vi "CS-4 Get Rates.vi"(6 "error in (no error)":errorcluster, 9 "VISA session":refnum<visa-resource-name>) -> (0 "error out":errorcluster, 2 "sweep rates":T1={"rate 0"=0.5, "rate 1"=0.25, "rate 2"=0.1, "rate 3"=10.0} {"rate 3" min=0.0 max=100.0 step=1.0 format="%.4f"; "rate 2" min=0.0 max=100.0 step=0.05 format="%.4f"; "rate 1" min=0.0 max=100.0 step=0.05 format="%.4f"; "rate 0" min=0.0 max=100.0 step=0.05 format="%.4f"}, 3 "dup VISA session":refnum<visa-resource-name>)   [LabVIEW 2016]
doc: "CS-4 Get Ratess.vi will return the sweep rates for each sweep range and for the fast sweep mode."
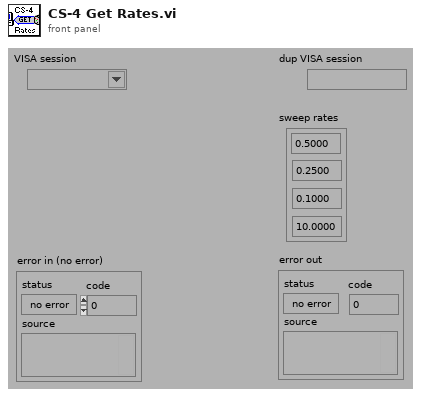
[diagram p1: front panel]
types:
  T1 = cluster{"rate 0":dbl, "rate 1":dbl, "rate 2":dbl, "rate 3":dbl}
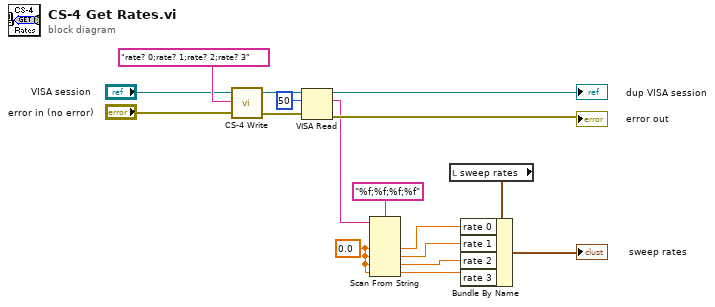
[diagram p0: block diagram]
diagram:
  w5 = 0.0
  n1 = call "CS-4 Write.vi"("error in (no error)"="error in (no error)", "write buffer (\"\")"="rate? 0;rate? 1;rate? 2;rate? 3", "VISA session"="VISA session") -> ("error out"=w10:errorcluster, "dup VISA session"=w11:refnum<visa-resource-name>)  [unwired: 1 out]
  n2 = VISA Read(VISA resource name=w11, byte count=u32 50 ("byte count (0)"), error in (no error)=w10) -> (VISA resource name out=→"dup VISA session":refnum<visa-resource-name>, read buffer=w6:string, error out=→"error out":errorcluster)  [unwired: 1 out]
  n3 = Scan From String(format string="%f;%f;%f;%f", input string=w6, default 1=w5, default 2=w5, default 3=w5, default 4=w5) -> (output 1=w4:dbl, output 2=w3:dbl, output 3=w2:dbl, output 4=w1:dbl)  [unwired: 2 in, 3 out]
  n4 = local read "sweep rates"() -> (w9:T1)
  n5 = Bundle By Name(cluster=w9, "rate 0"=w4, "rate 1"=w3, "rate 2"=w2, "rate 3"=w1) -> (→"sweep rates":T1)
